vi "meTEC_Create Error Cluster.vi"(8 "error in (no error)":errorcluster, 9 "Error Parameter":string, 10 "Error Instance":string, 11 "Error Number":string) -> (0 "error out":errorcluster)   [LabVIEW 2010]
panel:
  # "--- Outputs ---"
  # "--- Inputs ---"
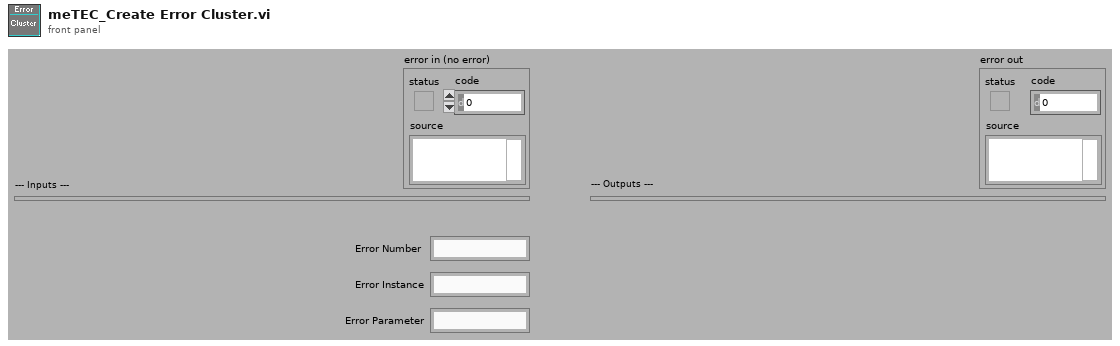
[diagram p1: front panel]
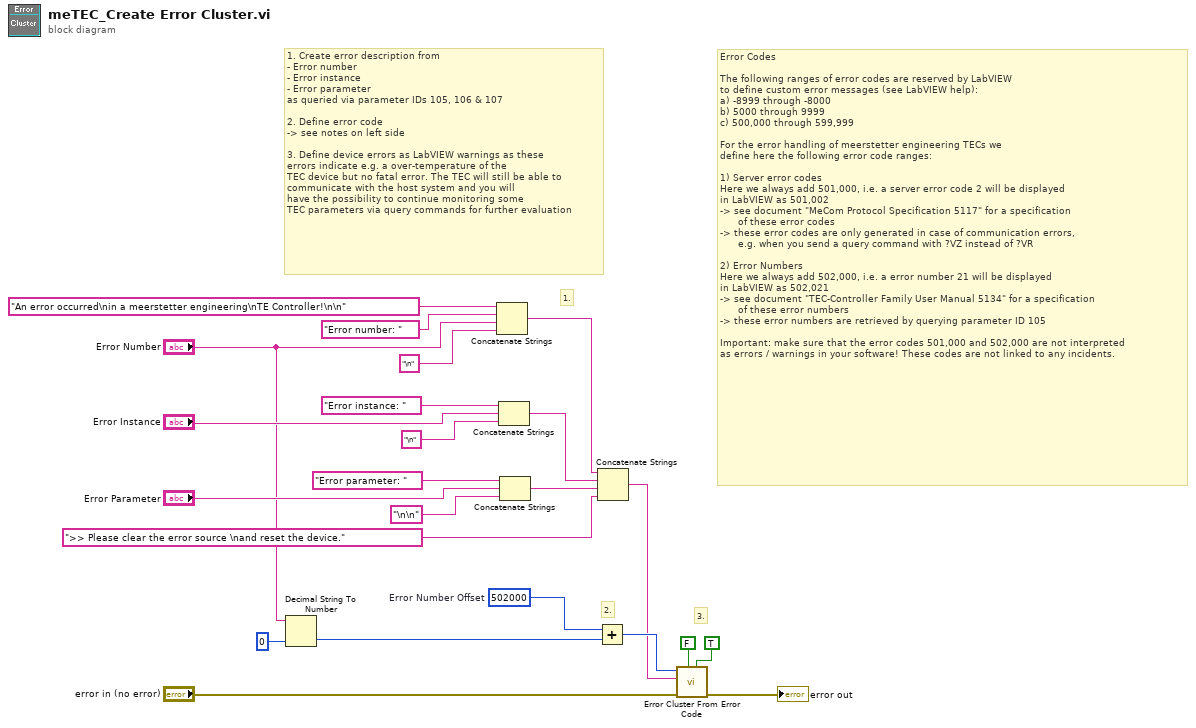
[diagram p0: block diagram]
diagram:
  w11 = 502000  # Error Number Offset
  # "3."
  # "Error Codes\n\nThe following ranges of error codes are reserved by LabVIEW\nto define custom error messages (see LabVIEW help):\na) -8999 through -8000 \nb) 5000 through 9999 \nc) 500,000 through 599,999\n\nFor the error handling of meerstetter engineering TECs we\ndefine here the following error code ranges:\n\n1) Server error codes\nHere we always add 501,000, i.e. a server error code 2 will be displayed\nin LabVIEW as 501,002\n-> see document \"MeCom Protocol Specification 5117\" for a specification \n      of these error codes\n-> these error codes are only generated in case of communication errors, \n      e.g. when you send a query command with ?VZ instead of ?VR \n\n2) Error Numbers\nHere we always add 502,000, i.e. a error number 21 will be displayed\nin LabVIEW as 502,021 \n-> see document \"TEC-Controller Family User Manual 5134\" for a specification \n      of these error numbers\n-> these error numbers are retrieved by querying parameter ID 105 \n\nImportant: make sure that the error codes 501,000 and 502,000 are not interpreted\nas errors / warnings in your software! These codes are not linked to any incidents."
  # "2."
  # "1."
  # "1. Create error description from\n- Error number\n- Error instance\n- Error parameter\nas queried via parameter IDs 105, 106 & 107\n\n2. Define error code\n-> see notes on left side\n\n3. Define device errors as LabVIEW warnings as these\nerrors indicate e.g. a over-temperature of the \nTEC device but no fatal error. The TEC will still be able to \ncommunicate with the host system and you will \nhave the possibility to continue monitoring some \nTEC parameters via query commands for further evaluation"
  n1 = Decimal String To Number(string="Error Number", default (0L)=0 ("default (0 U32)")) -> (number=w4:i32)  [unwired: 1 in, 1 out]
  n2 = Concatenate Strings("An error occurred\nin a meerstetter engineering\nTE Controller!\n\n" ("string"), "Error number: " ("string"), "Error Number", "\n" ("string")) -> (w13:string)
  n3 = Concatenate Strings("Error instance: " ("string"), "Error Instance", "\n" ("string")) -> (w14:string)
  n4 = Concatenate Strings("Error parameter: " ("string"), "Error Parameter", "\n\n" ("string")) -> (w15:string)
  n5 = Add(x=w11, y=w4) -> (x+y=w22:i32)
  n6 = Concatenate Strings(w13, w14, w15, ">> Please clear the error source \nand reset the device." ("string")) -> (w12:string)
  n7 = call <vilib>:"Error Cluster From Error Code.vi"("is warning? (False)"=TRUE, "show call chain? (False)"=FALSE, "error in (no error)"="error in (no error)", "error message (\"\")"=w12, "error code (0)"=w22) -> ("error out"=→"error out":errorcluster)  [unwired: 4 in]
